vi "Read PID configuration.vi"(8 "error in (no error)":errorcluster, 11 "PID Control in":refnum<class "PID Control.lvclass">) -> (0 "error out":errorcluster, 2 "PID configuration":T1, 3 "PID Control out":refnum<class "PID Control.lvclass">)   [LabVIEW 2016, in "PID Control.lvclass"]
uses:
  PID Control.lvclass
  PID Configuration.ctl
  PID Control.lvclass/PID Control.ctl
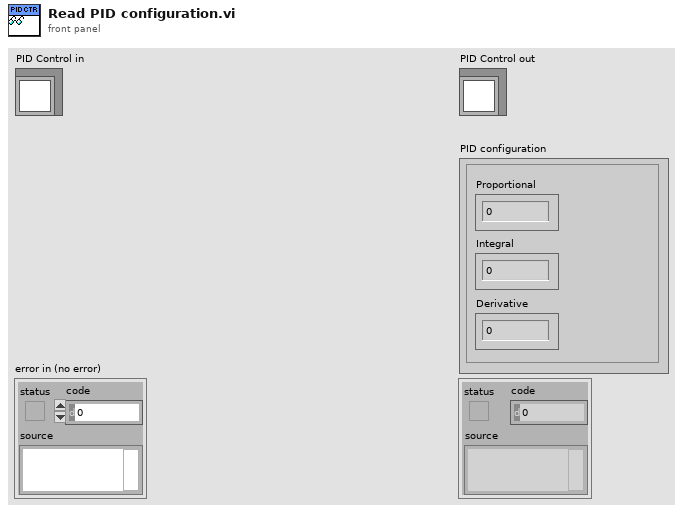
[diagram p1: front panel]
types:
  T1 = typedef "PID Configuration.ctl" = cluster{"Proportional":dbl, "Integral":dbl, "Derivative":dbl}
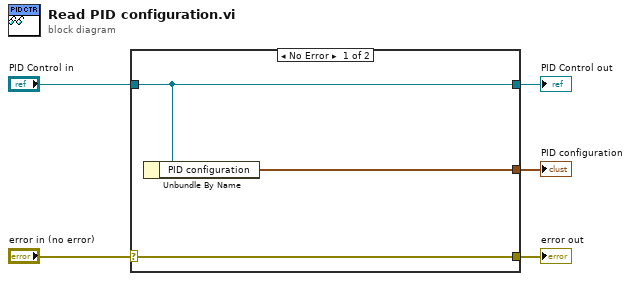
[diagram p0: block diagram]
diagram:
  n1 = case shown="No Error" "error in (no error)" {
    selector: "error in (no error)" -> [w8 w9]
    tunnel: [w8 w9] -> w4
    tunnel: [w7 w10] -> w2
    tunnel: "PID Control in" -> [w7 w10]
    tunnel: [w6 _] -> w1
    frame No Error {
      n2 = Unbundle By Name(w7) -> ("PID configuration"=w6:T1)
    }
    frame Error {
    }
  }
  "error out" <- w4
  "PID Control out" <- w2
  "PID configuration" <- w1
